vi "Close Path Associated Instruments.vi"(0 "Path Groups in":refnum<class "Path Group.lvclass">[](array[class]), 11 "error in (no error)":errorcluster) -> (4 "Path Groups out":refnum<class "Path Group.lvclass">[](array[class]), 15 "error out":errorcluster)   [LabVIEW 2023, in "RFCalAndFixtureCharact.Common.lvlib"]
uses:
  RFCalAndFixtureCharact.Common.lvlib
  Base Classes/Path Group/Path Group.lvclass
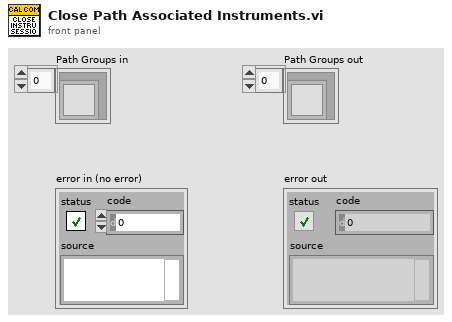
[diagram p1: front panel]
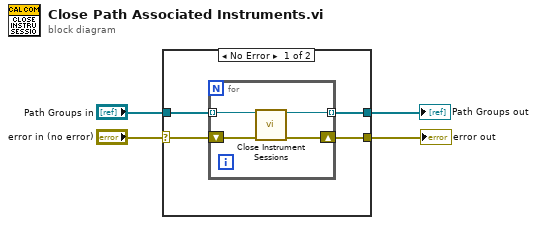
[diagram p0: block diagram]
diagram:
  n1 = case shown="No Error" "error in (no error)" {
    selector: "error in (no error)" -> [w8 w14]
    tunnel: [w6 w14] -> w3
    tunnel: "Path Groups in" -> [w7 w13]
    tunnel: [w5 w13] -> w1
    frame No Error {
      n2 = for {
        tunnel: w7 -> [w10] mode=indexing
        shift-right: [w11] -> w6
        shift-left: w8 -> [w12]
        tunnel: [w9] -> w5 mode=indexing
        n3 = call-dynamic "Close Instrument Sessions.vi"("Path Group in"=w10, "error in (no error)"=w12) -> ("Path Group out"=w9:refnum<class "Path Group.lvclass">, "error out"=w11:errorcluster)  [unwired: 12 in]
      }
    }
    frame Error {
    }
  }
  "error out" <- w3
  "Path Groups out" <- w1
